vi "DeCoF integer set.vi"(4 "error in":errorcluster, 5 "value":i32, 6 "param-name":string, 7 "Conncection ID in":T1) -> (0 "error out":errorcluster, 3 "Conncection ID out":T1)   [LabVIEW 2013]
uses:
  subVIs/DeCoF connection.ctl
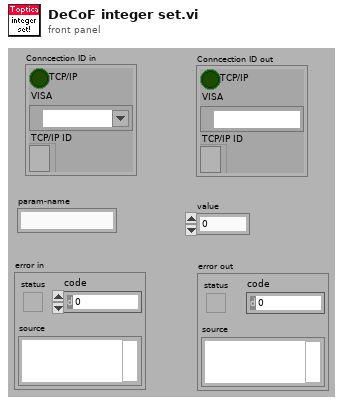
[diagram p1: front panel]
types:
  T1 = typedef "DeCoF connection.ctl" = cluster{"TCP/IP":bool, "VISA":refnum<visa-resource-name>, "TCP/IP ID":refnum<k5>}
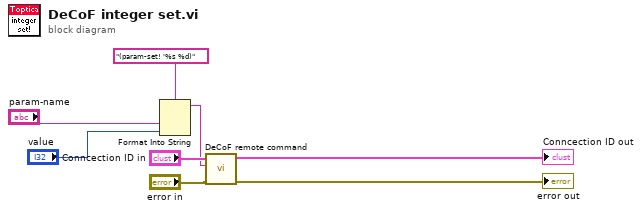
[diagram p0: block diagram]
diagram:
  n1 = Format Into String(format string="(param-set! '%s %d)", "param-name", "value") -> (resulting string=w3:string)  [unwired: 2 in, 1 out]
  n2 = call "DeCoF remote command.vi"("error in (no error)"="error in", "command"=w3, "Conncection ID in"="Conncection ID in") -> ("error out"=→"error out":errorcluster, "Conncection ID out"=→"Conncection ID out":T1)  [unwired: 2 in, 3 out]
